vi "RT Thermocouple.vi"(11 "Queue ref":T1) -> ()   [LabVIEW 2022 SP3]
uses:
  RT Controls/RT All Queue.ctl
  RT Controls/RT DAQ case.ctl
  RT Controls/RT All Loop Status.ctl
  <vilib>/DAQmx/read.llb/DAQmx Read (Analog 1D Wfm NChan NSamp).vi
  RT Create Task/RT TC Create Task.vi
  <vilib>/DAQmx/configure/timing.llb/DAQmx Timing (Sample Clock).vi
  RT Sub VI's/RT Global.vi
  <vilib>/DAQmx/miscellaneous.llb/DAQmx Fill In Error Info.vi
panel:
  out "overflow?":bool
  # "TC channel list"
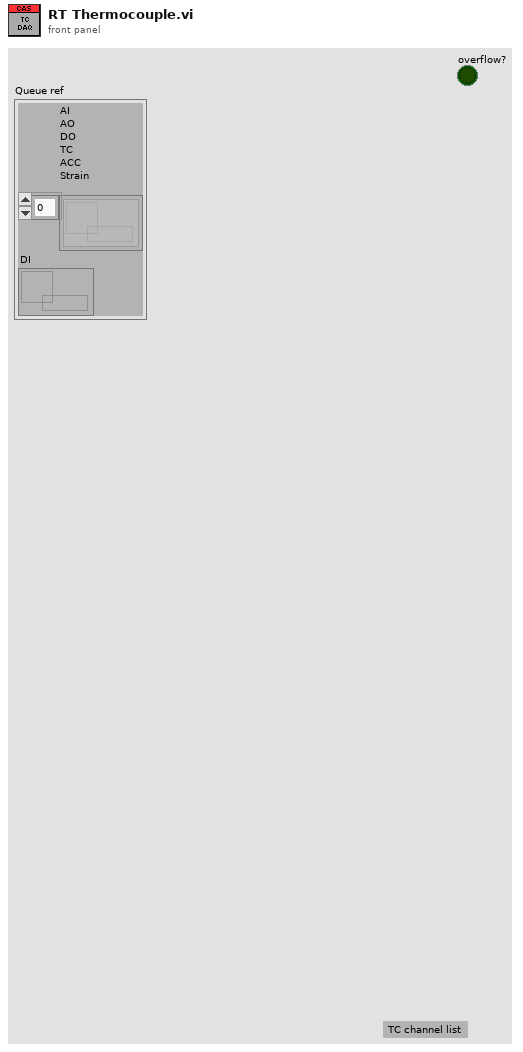
[diagram p1: front panel]
types:
  T1 = typedef "RT All Queue.ctl" = cluster{"AI\nAO\nDO\nTC\nACC\nStrain":refnum<queue>[], "DI":refnum<queue>}
  T2 = cluster{"in progress?":bool, "Start DAQ":refnum<notifier>, "task out":refnum<k21>, "TC Ref":refnum<queue>, "SPC":i32}
  T3 = typedef "RT DAQ case.ctl" = enum16{"Initailise", "Create Task", "Polevent", "Acquire", "Stop DAQ", "Error", "Exit"}
  T4 = typedef "RT All Loop Status.ctl" = enum16{"AI", "AO", "DI", "DO", "TC", "Strain", "ACC", "RT", "Log"}
  T5 = enum16{"Init", "Read 'All'", "Read 'n'", "Read '1'", "Write '1'", "Write 'n'", "Write 'All'"}
  T6 = typedef "RT All Notifer.ctl" = cluster{"Start DAQ":refnum<notifier>}
  T7 = cluster{"Analog input":bool, "Analog Output":bool, "Digital input":bool, "Digital output":bool, "Thermocouple":bool, "Strain Gauge":bool, "Accelerometer":bool}
  T8 = typedef "RT Config.ctl" = cluster{"AO config":cluster{"Channel_Name":string, "Channel_Number":string, "Default_Value":dbl, "Units":string}[], "AI config":cluster{"Channel_Name":string, "Channel_Number":string, "Pre_Scale_min":dbl, "Pre_Scale_max":dbl, "Sensor_min":dbl, "Sensor_max":dbl, "Units":string}[], "DI config":cluster{"Channel_Name":string, "Channel_Number":string, "Default_Value":bool, "Units":bool}[], "DO config":cluster{"Channel_Name":string, "Channel_Number":string, "Default_Value":bool, "Units":bool}[], "TC config":cluster{"Channel_Name":string, "Channel_Number":string, "Pre_Scale_min":dbl, "Pre_Scale_max":dbl, "units":i32, " type":i32}[], "ACC config":cluster{"Channel_Name":string, "Channel_Number":string, "Pre_Scale_min":dbl, "Pre_Scale_max":dbl, "Terminal configuration":i32, "Sensitivity":dbl, "Sensitivity units":i32}[], "SG config":cluster{"Channel_Name":string, "Channel_Number":string, "Pre_Scale_min":dbl, "Pre_Scale_max":dbl}[], "Strain Gauge Settings":cluster{"poisson ratio":dbl, "nominal gage resistance":dbl, "gage factor":dbl}, "Bridge Settings ":cluster{"strain configuration":i32, "lead wire resistance":dbl, "initial bridge voltage":dbl, "voltage excitation source":i32, "voltage excitation value":dbl}, "Sample Rate":cluster{"AI Sample Rate":dbl, "AO Sample Rate":dbl, "DI Sample Rate":dbl, "TC Sample Rate":dbl, "DO Sample Rate":dbl, "SG Sample Rate":dbl, "ACC Sample Rate":dbl}}
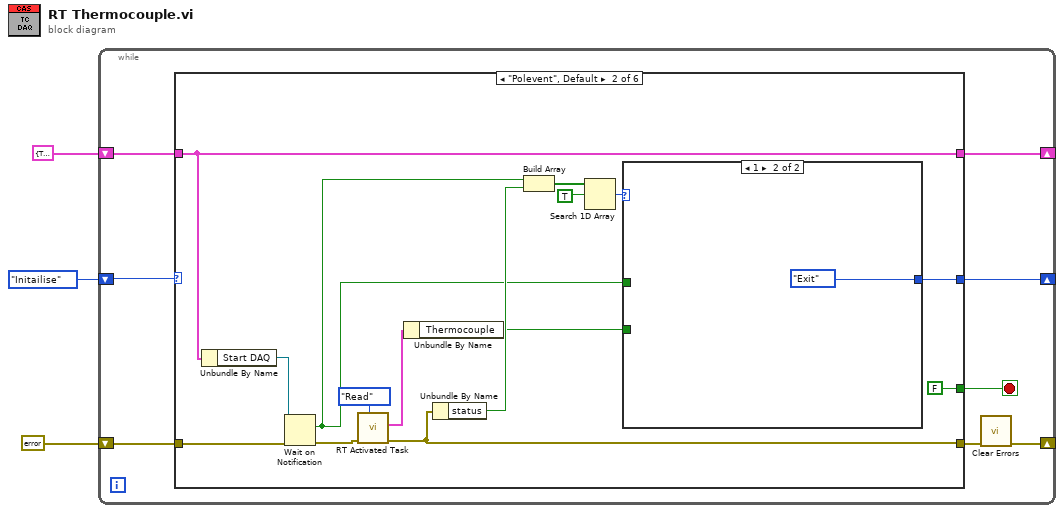
[diagram p0: block diagram]
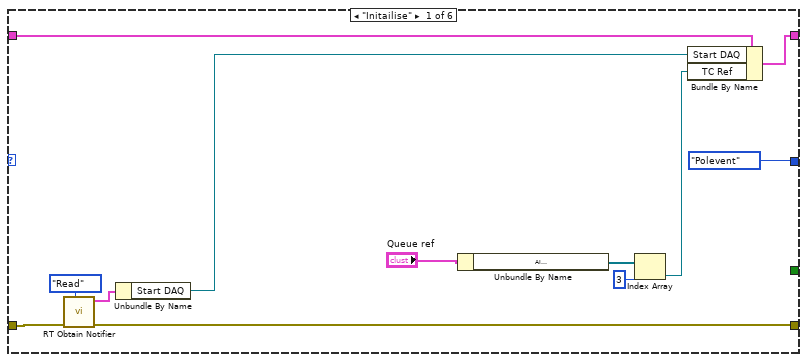
[diagram p2: hidden frame]
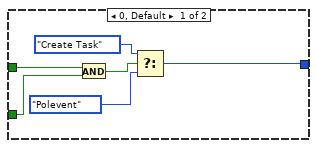
[diagram p3: hidden frame]
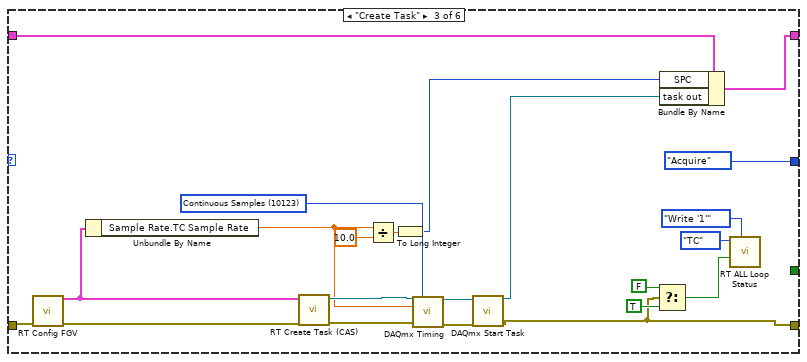
[diagram p4: hidden frame]
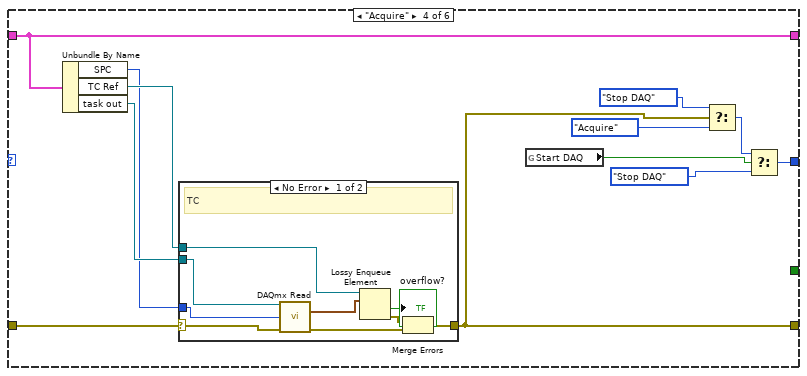
[diagram p5: hidden frame]
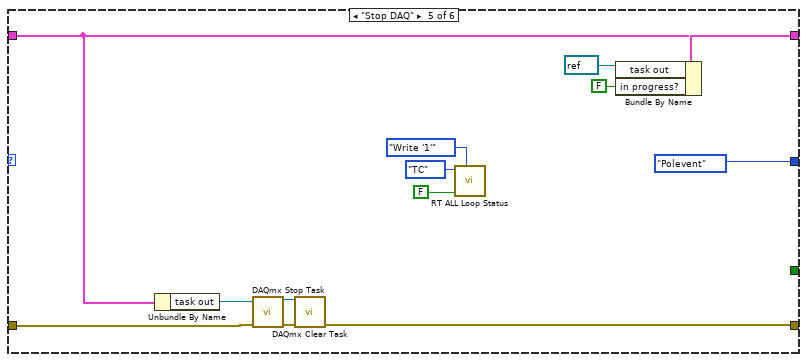
[diagram p7: hidden frame]
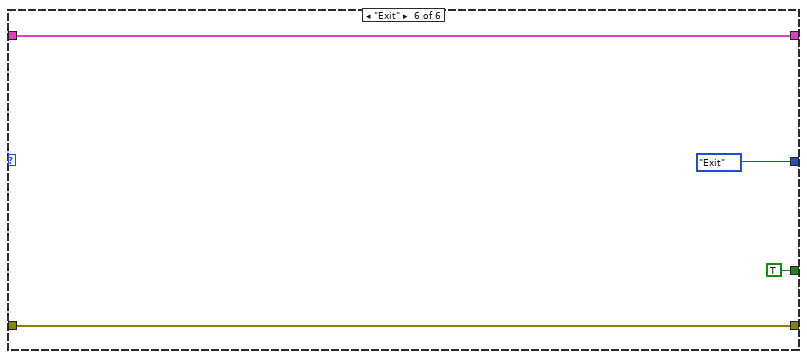
[diagram p8: hidden frame]
diagram:
  n1 = while {
    shift-right: [w4] -> _
    shift-left: errorcluster {"status"=FALSE, "code"=0, "source"=""} ("error out") -> [w10]
    shift-right: [w8] -> _
    shift-left: T2 {"in progress?"=TRUE, "Start DAQ"=refnum, "task out"="", "TC Ref"=refnum, "SPC"=0} -> [w9]
    shift-right: [w7] -> _
    shift-left: RT_DAQ_case."Initailise" -> [w6]
    stop <- w11 stop-if-true
    n2 = case shown="\"Polevent\", Default" w6 {
      tunnel: [_ FALSE _ _ _ TRUE] -> w11
      tunnel: w10 -> [w14 w28 w57 w76 w96 w106]
      tunnel: [w13 w24 w60 w70 w97 w106] -> w5
      tunnel: w9 -> [w23 w36 w67 w77 w101 w105]
      tunnel: [w21 w36 w66 w77 w102 w105] -> w8
      tunnel: [RT_DAQ_case."Polevent" w37 RT_DAQ_case."Acquire" w78 RT_DAQ_case."Polevent" RT_DAQ_case."Exit"] -> w7
      frame "Initailise" {
        n3 = call "RT Obtain Notifier.vi"("Case"=enum16{"Obtain", "Read"}."Read", "error in (no error)"=w14) -> ("error out"=w13:errorcluster, "All Notifier"=w12:T6)  [unwired: 8 in]
        n4 = Unbundle By Name(w12) -> ("Start DAQ"=w22:refnum<notifier>)
        n5 = Unbundle By Name("Queue ref") -> ("AI\nAO\nDO\nTC\nACC\nStrain"=w19:refnum<queue>[])
        n6 = Index Array(array=w19, index=3) -> (element=w18:refnum<queue>)
        n7 = Bundle By Name(cluster=w23, "Start DAQ"=w22, "TC Ref"=w18) -> (w21:T2)
      }
      frame "Polevent", Default {
        n8 = Unbundle By Name(w36) -> ("Start DAQ"=w35:refnum<notifier>)
        n9 = Wait on Notification(notifier=w35, error in (no error)=w28) -> (notification=w29:bool, error out=w25:errorcluster)  [unwired: 2 in, 2 out]
        n10 = call "RT Activated Task.vi"("Enum"=enum16{"Read", "Write"}."Read", "error in (no error)"=w25) -> ("error out"=w24:errorcluster, "Activate Task 2"=w27:T7)  [unwired: 7 in, 1 out]
        n11 = Unbundle By Name(w27) -> ("Thermocouple"=w30:bool)
        n12 = Unbundle By Name(w24) -> ("status"=w34:bool)
        n13 = Build Array(w29, w34) -> (w33:bool[])
        n14 = Search 1D Array(1D array=w33, element=TRUE) -> (index of element=w31:i32)  [unwired: 1 in]
        n15 = case shown="1" w31 {
          tunnel: [w44 RT_DAQ_case."Exit"] -> w37
          tunnel: w30 -> [w42 _]
          tunnel: w29 -> [w41 _]
          frame 0, Default {
            n16 = And(x=w41, y=w42) -> (x .and. y?=w43:bool)
            n17 = Select(t=RT_DAQ_case."Create Task", s=w43, f=RT_DAQ_case."Polevent") -> (s? t:f=w44:T3)
          }
          frame 1 {
          }
        }
      }
      frame "Create Task" {
        w65 = 10123 items=["Finite Samples"=10178, "Continuous Samples"=10123, "Hardware Timed Single Point"=12522] ("sample mode")
        n18 = call "RT Config FGV.vi"("error in (no error)"=w57) -> ("error out"=w56:errorcluster, "Data out"=w50:T8)  [unwired: 9 in]
        n19 = Unbundle By Name(w50) -> ("Sample Rate.TC Sample Rate"=w49:dbl)
        n20 = call-poly "RT Create Task (CAS).vi"("error in"=w56, "config"=w50) -> ("error out"=w55:errorcluster, "task out"=w54:refnum<k21>)  [unwired: 7 in, 1 out]
        n21 = Divide(x=w49, y=10.0) -> (x/y=w47:dbl)
        n22 = To Long Integer(number=w47) -> (32bit integer=w46:i32)
        n23 = call-poly <vilib>:"DAQmx Timing.vi"("task/channels in"=w54, "sample mode"=w65, "rate"=w49, "error in"=w55) -> ("task out"=w62:refnum<k21>, "error out"=w61:errorcluster)  [unwired: 10 in]
        n24 = call <vilib>:"DAQmx Start Task.vi"("task/channels in"=w62, "error in"=w61) -> ("task out"=w59:refnum<k21>, "error out"=w60:errorcluster)  [unwired: 12 in]
        n25 = Select(t=FALSE, s=w60, f=TRUE) -> (s? t:f=w51:bool)
        n26 = Bundle By Name(cluster=w67, "SPC"=w46, "task out"=w59) -> (w66:T2)
        n27 = call "RT ALL Loop Status.vi"("Option"=T5."Write '1'", "Status"=w51, "Loop"=RT_All_Loop_Status."TC") -> ()  [unwired: 6 in, 3 out]
      }
      frame "Acquire" {
        n28 = Unbundle By Name(w77) -> ("SPC"=w68:i32, "TC Ref"=w75:refnum<queue>, "task out"=w74:refnum<k21>)
        n29 = case shown="No Error" w76 {
          selector: w76 -> [w84 w89]
          tunnel: w74 -> [w83 _]
          tunnel: [w86 w89] -> w70
          tunnel: w75 -> [w85 _]
          tunnel: w68 -> [w80 _]
          frame No Error {
            # "TC"
            n30 = call-poly <vilib>:"DAQmx Read.vi"("task/channels in"=w83, "number of samples per channel"=w80, "error in"=w84) -> ("data"=w82:waveform(dbl)[], "error out"=w87:errorcluster)  [unwired: 10 in, 1 out]
            n31 = Lossy Enqueue Element(queue=w85, element=w82) -> (overflow?=→"overflow?":bool, error out=w88:errorcluster)  [unwired: 1 in, 2 out]
            n32 = Merge Errors(w88, w87) -> (w86:errorcluster)
          }
          frame Error {
          }
        }
        n33 = global read "RT Global.vi" "Start DAQ"() -> (w69:bool)
        n34 = Select(t=RT_DAQ_case."Stop DAQ", s=w70, f=RT_DAQ_case."Acquire") -> (s? t:f=w79:T3)
        n35 = Select(t=w79, s=w69, f=RT_DAQ_case."Stop DAQ") -> (s? t:f=w78:T3)
      }
      frame "Stop DAQ" {
        n36 = Unbundle By Name(w101) -> ("task out"=w95:refnum<k21>)
        n37 = call <vilib>:"DAQmx Stop Task.vi"("task/channels in"=w95, "error in"=w96) -> ("task out"=w94:refnum<k21>, "error out"=w98:errorcluster)  [unwired: 12 in]
        n38 = call <vilib>:"DAQmx Clear Task.vi"("task in"=w94, "error in"=w98) -> ("error out"=w97:errorcluster)  [unwired: 13 in]
        n39 = call "RT ALL Loop Status.vi"("Option"=T5."Write '1'", "Status"=FALSE, "Loop"=RT_All_Loop_Status."TC") -> ()  [unwired: 6 in, 3 out]
        n40 = Bundle By Name(cluster=w101, "task out"=refnum<k21> refnum, "in progress?"=FALSE) -> (w102:T2)
      }
      frame "Exit" {
      }
    }
    n41 = call <vilib>:"Clear Errors.vi"("error in (no error)"=w5) -> ("error out"=w4:errorcluster)  [unwired: 5 in, 1 out]
  }
